vi "Calculate Pace Amp_backup.vi"(8 "Pace Waveform":waveform(dbl), 9 "波形图":waveform(dbl)[](array[waveform])=[{"t0"=timestamp(3440194019.9959836 s since 1904-01-01), "dt"=1.9999999999999944e-06, "Y"=array[49999 elements], "attributes"=variant("NI_ChannelName"=variant(string "6259A/ai15"), "NI_UnitDescription"=variant(string "Volts"))}, {"t0"=timestamp(3440194019.9959836 s since 1904-01-01), "dt"=1.9999999999999944e-06, "Y"=array[49999 elements], "attributes"=variant("NI_ChannelName"=variant(string "6259A/ai21"), "NI_UnitDescription"=variant(string "Volts"))}], 10 "设定脉宽":dbl, 11 "设置的起搏幅度":dbl=4.0) -> (0 "PW":dbl, 1 "Vpgb（起搏幅度） 国标1":dbl, 2 "VP （200u（起搏幅度））":dbl, 3 "VP max":dbl, 4 "Vpgb/vh":dbl, 5 "TE":dbl, 6 "VP/vh":dbl, 7 "LE":dbl)   [LabVIEW 2016]
panel:
  out "b":dbl
  out "k":dbl
  out "element":dbl
  out "dt":dbl
  out "Waveform Graph":waveform(dbl)(graph)
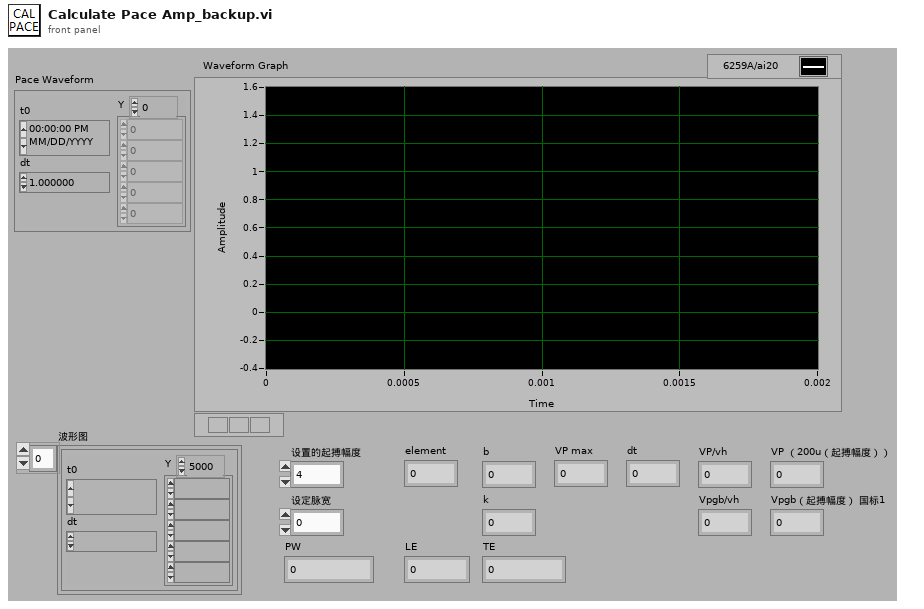
[diagram p1: front panel]
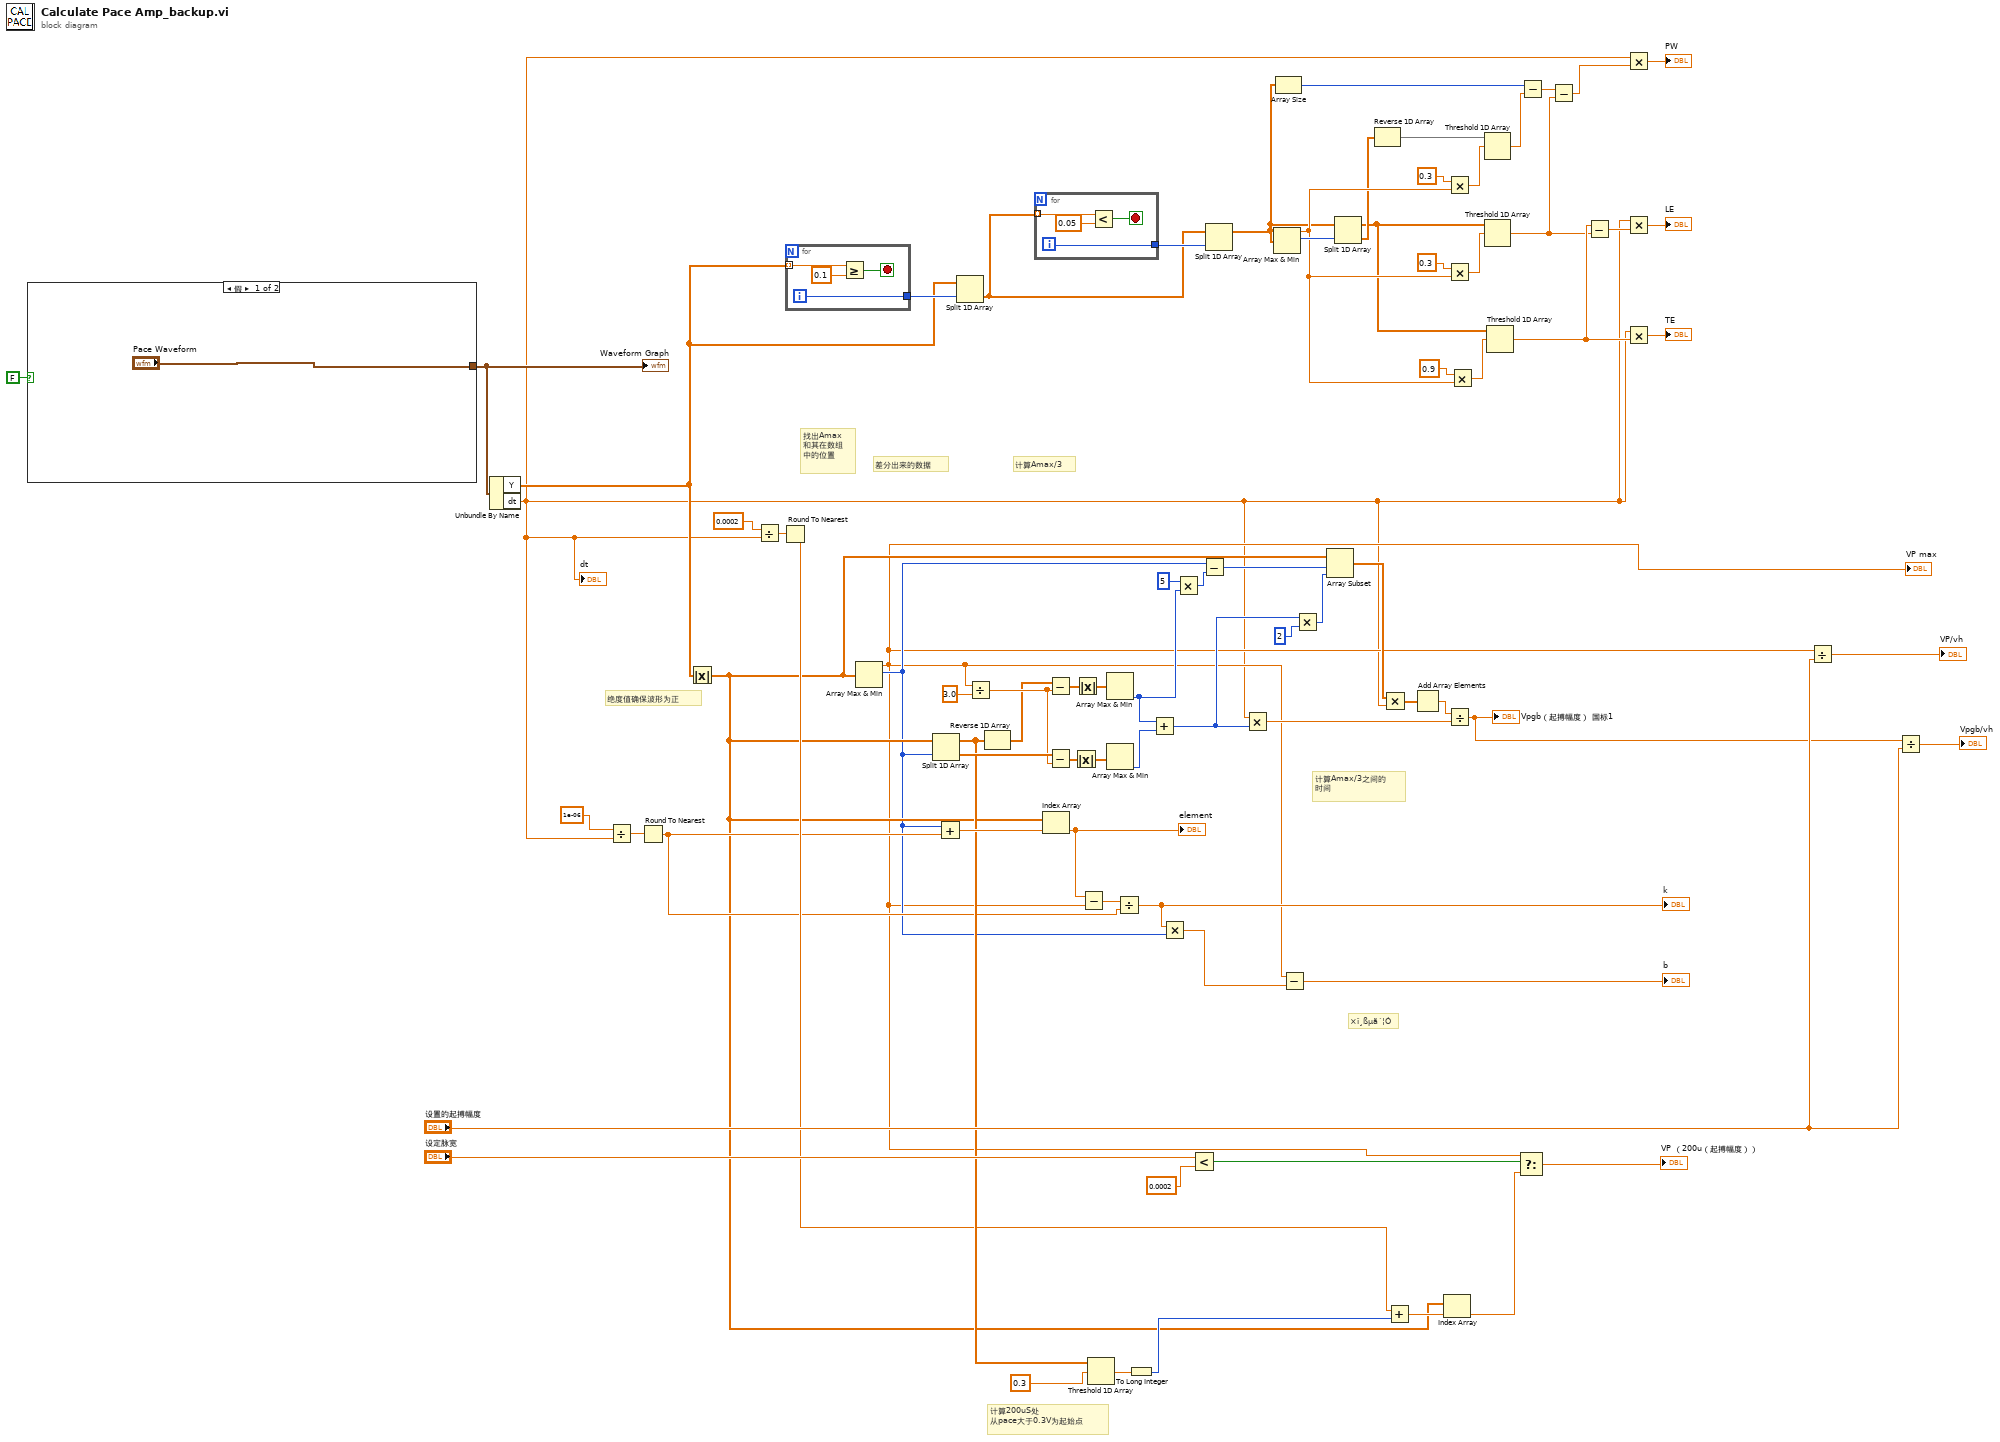
[diagram p0: block diagram]
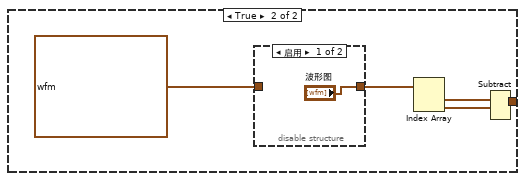
[diagram p2: hidden frame]
diagram:
  # "计算Amax/3之间的\n时间"
  # "计算Amax/3"
  # "找出Amax\n和其在数组\n中的位置"
  # "×î¸ßµã´¦Ó"
  # "绝度值确保波形为正"
  # "计算200uS处\n从pace大于0.3V为起始点"
  # "差分出来的数据"
  n1 = case shown="假" FALSE {
    tunnel: ["Pace Waveform" w80] -> w40
    frame False {
    }
    frame True {
      n2 = disable-structure shown="启用" {
        disable-tunnel: ["波形图" w86] -> w83
        disable-tunnel: waveform(dbl)[] [{"t0"=timestamp(3440384625.714352 s since 1904-01-01), "dt"=1.9999999999999944e-06, "Y"=array[49999 elements], "attributes"=variant("NI_ChannelName"=variant(string "6259A/ai17"), "NI_UnitDescription"=variant(string "Volts"))}, {"t0"=timestamp(3440384625.714352 s since 1904-01-01), "dt"=1.9999999999999944e-06, "Y"=array[49999 elements], "attributes"=variant("NI_ChannelName"=variant(string "6259A/ai20"), "NI_UnitDescription"=variant(string "Volts"))}] ("波形图 2") -> [_ w86]
        frame Enabled {
        }
        frame Disabled {
        }
      }
      n3 = Index Array(array=w83) -> (element #1=w84:waveform(dbl), element #2=w81:waveform(dbl))  [unwired: 2 in]
      n4 = Subtract(1:w81, 2:w84) -> (0:w80:waveform(dbl))  [unwired: 1 in, 1 out]
    }
  }
  "Waveform Graph" <- w40
  n5 = Unbundle By Name(w40) -> ("Y"=w25:dbl[], "dt"=w4:dbl)
  "dt" <- w4
  n6 = Divide(x=1e-06 ("dt 2"), y=w4) -> (x/y=w63:dbl)
  n7 = Round To Nearest(number=w63) -> (nearest integer value=w32:dbl)
  n8 = Absolute Value(x=w25) -> (abs(x)=w31:dbl[])
  n9 = Divide(x=0.0002 ("dt 2"), y=w4) -> (x/y=w77:dbl)
  n10 = Round To Nearest(number=w77) -> (nearest integer value=w34:dbl)
  n11 = for {
    tunnel: w25 -> [w90] mode=indexing
    tunnel: [w87] -> w28
    i -> [w87]
    stop <- w88 stop-if-true
    n12 = Greater Or Equal?(x=w90, y=0.1) -> (x >= y?=w88:bool)
  }
  n13 = Array Max & Min(array=w31) -> (max value=w29:dbl, max index (indices)=w30:i32)  [unwired: 2 out]
  "VP max" <- w29
  n14 = Split 1D Array(array=w31, index=w30) -> (first subarray=w39:dbl[], second subarray=w72:dbl[])
  n15 = Add(x=w30, y=w32) -> (x+y=w61:dbl)
  n16 = Split 1D Array(array=w25, index=w28) -> (second subarray=w26:dbl[])  [unwired: 1 out]
  n17 = Divide(x=w29, y=3.0) -> (x/y=w71:dbl)
  n18 = Reverse 1D Array(array=w39) -> (reversed array=w52:dbl[])
  n19 = for {
    tunnel: w26 -> [w94] mode=indexing
    tunnel: [w91] -> w27
    i -> [w91]
    stop <- w92 stop-if-true
    n20 = Less?(x=w94, y=0.05) -> (x < y?=w92:bool)
  }
  n21 = Index Array(array=w31, index=w61) -> (element=w51:dbl)
  "element" <- w51
  n22 = Subtract(x=w52, y=w71) -> (x-y=w70:dbl[])
  n23 = Subtract(x=w72, y=w71) -> (x-y=w69:dbl[])
  n24 = Absolute Value(x=w69) -> (abs(x)=w67:dbl[])
  n25 = Absolute Value(x=w70) -> (abs(x)=w68:dbl[])
  n26 = Subtract(x=w51, y=w29) -> (x-y=w60:dbl)
  n27 = Threshold 1D Array(2:0.3 ("y"), 3:w39) -> (0:w37:dbl)  [unwired: 1 in]
  n28 = Array Max & Min(array=w68) -> (min index (indices)=w48:i32)  [unwired: 3 out]
  n29 = Array Max & Min(array=w67) -> (min index (indices)=w66:i32)  [unwired: 3 out]
  n30 = Divide(x=w60, y=w32) -> (x/y=w58:dbl)
  "k" <- w58
  n31 = To Long Integer(number=w37) -> (32bit integer=w36:i32)
  n32 = Add(x=w48, y=w66) -> (x+y=w45:i32)
  n33 = Multiply(x=w58, y=w30) -> (x*y=w59:dbl)
  n34 = Multiply(x=5, y=w48) -> (x*y=w46:i32)
  n35 = Less?(x="设定脉宽", y=0.0002 ("dt 2")) -> (x < y?=w54:bool)
  n36 = Subtract(x=w30, y=w46) -> (x-y=w43:i32)
  n37 = Split 1D Array(array=w26, index=w27) -> (first subarray=w5:dbl[])  [unwired: 1 out]
  n38 = Multiply(x=w4, y=w45) -> (x*y=w49:dbl)
  n39 = Array Max & Min(array=w5) -> (max value=w6:dbl, max index (indices)=w13:i32)  [unwired: 2 out]
  n40 = Array Size(array=w5) -> (size(s)=w20:i32)
  n41 = Subtract(x=w29, y=w59) -> (x-y=→"b":dbl)
  n42 = Multiply(x=w45, y=2) -> (x*y=w42:i32)
  n43 = Array Subset(array=w31, index=w43, length=w42) -> (w41:dbl[])
  n44 = Split 1D Array(array=w5, index=w13) -> (first subarray=w2:dbl[], second subarray=w3:dbl[])
  n45 = Reverse 1D Array(array=w3) -> (reversed array=w9:dbl[])
  n46 = Multiply(x=w41, y=w4) -> (x*y=w65:dbl[])
  n47 = Add(x=w34, y=w36) -> (x+y=w53:dbl)
  n48 = Add Array Elements(numeric array=w65) -> (sum=w50:dbl)
  n49 = Index Array(array=w31, index=w53) -> (element=w33:dbl)
  n50 = Multiply(x=0.3, y=w6) -> (x*y=w10:dbl)
  n51 = Multiply(x=0.3, y=w6) -> (x*y=w23:dbl)
  n52 = Divide(x=w50, y=w49) -> (x/y=w64:dbl)
  "Vpgb（起搏幅度） 国标1" <- w64
  n53 = Multiply(x=0.9, y=w6) -> (x*y=w21:dbl)
  n54 = Threshold 1D Array(2:w10, 3:w9) -> (0:w8:dbl)  [unwired: 1 in]
  n55 = Threshold 1D Array(2:w23, 3:w2) -> (0:w7:dbl)  [unwired: 1 in]
  n56 = Threshold 1D Array(2:w21, 3:w2) -> (0:w12:dbl)  [unwired: 1 in]
  n57 = Select(t=w29, s=w54, f=w33) -> (s? t:f=→"VP （200u（起搏幅度））":dbl)
  n58 = Subtract(x=w20, y=w8) -> (x-y=w19:dbl)
  n59 = Subtract(x=w19, y=w7) -> (x-y=w18:dbl)
  n60 = Subtract(x=w12, y=w7) -> (x-y=w14:dbl)
  n61 = Multiply(x=w4, y=w18) -> (x*y=→"PW":dbl)
  n62 = Multiply(x=w4, y=w14) -> (x*y=→"LE":dbl)
  n63 = Multiply(x=w4, y=w12) -> (x*y=→"TE":dbl)
  n64 = Divide(x=w29, y="设置的起搏幅度") -> (x/y=→"VP/vh":dbl)
  n65 = Divide(x=w64, y="设置的起搏幅度") -> (x/y=→"Vpgb/vh":dbl)
